vi "CaseStructure - Move Frame.vi"(8 "error in (no error)":errorcluster, 9 "New Position":i32, 10 "Current Position":i32, 11 "CaseStructure in":refnum<vi>) -> (0 "error out":errorcluster, 3 "CaseStructure out":refnum<vi>)   [LabVIEW 2020]
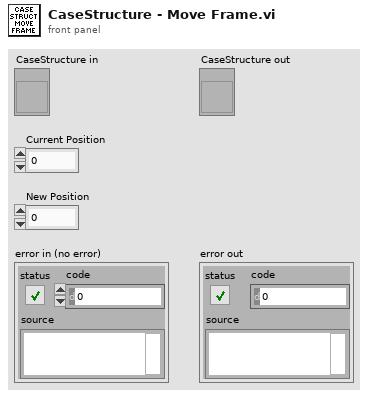
[diagram p1: front panel]
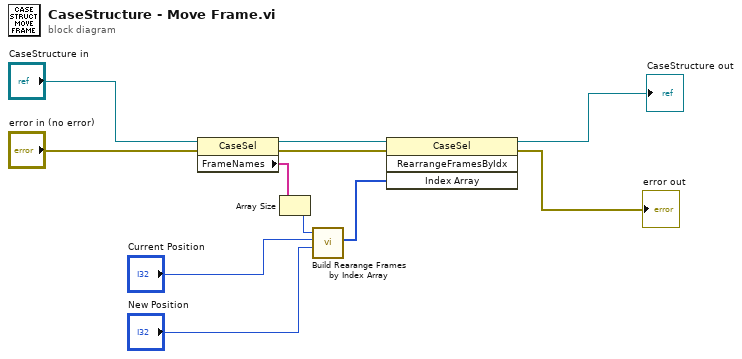
[diagram p0: block diagram]
diagram:
  n1 = property class="CaseSel"(reference="CaseStructure in", error in="error in (no error)") -> (reference out=w7:refnum<vi>, error out=w9:errorcluster, "FrameNames"=w10:string[])
  n2 = Array Size(array=w10) -> (size(s)=w2:i32)
  n3 = call "Build Rearange Frames by Index Array.vi"("New Position"="New Position", "Current Position"="Current Position", "N"=w2) -> ("New Positions Array"=w4:i32[])  [unwired: 8 in]
  n4 = invoke class="CaseSel" method="RearrangeFramesByIdx"(reference=w7, error in=w9, "Index Array"=w4) -> (reference out=→"CaseStructure out":refnum<vi>, error out=→"error out":errorcluster)  [unwired: 1 in, 2 out]
